vi "wheel velocities.vi"(6 "Track Width":dbl, 11 "Path Data":T1={"Path"=[], "Target Velocities"=[], "Robot Location"=[], "Relative Robot Angle (rad)"=0.0, "Curvature"=0.0, "Lookahead Point"=[3064.399009129367, 18229.833030071386], "Lookahead Index"=8.422809037111724, "Closest Point"=[], "Closest Point Index"=0, "Left Velocity"=0.0, "Right Velocity"=0.0, "Left Encoder Vel"=0, "Right Encoder Vel"=0, "Left Encoder Pos"=0, "Right Encoder Pos"=0, "Inital Robot Angle (deg)"=0.0}) -> (3 "Path Data":T1={"Path"=[], "Target Velocities"=[], "Robot Location"=[], "Relative Robot Angle (rad)"=0.0, "Curvature"=0.0, "Lookahead Point"=[3064.399009129367, 18229.833030071386], "Lookahead Index"=8.422809037111724, "Closest Point"=[], "Closest Point Index"=0, "Left Velocity"=0.0, "Right Velocity"=0.0, "Left Encoder Vel"=0, "Right Encoder Vel"=0, "Left Encoder Pos"=0, "Right Encoder Pos"=0, "Inital Robot Angle (deg)"=0.0})   [LabVIEW 2018]
uses:
  path data.ctl
panel:
  out "Right Velocity":dbl
  out "Left Velocity":dbl
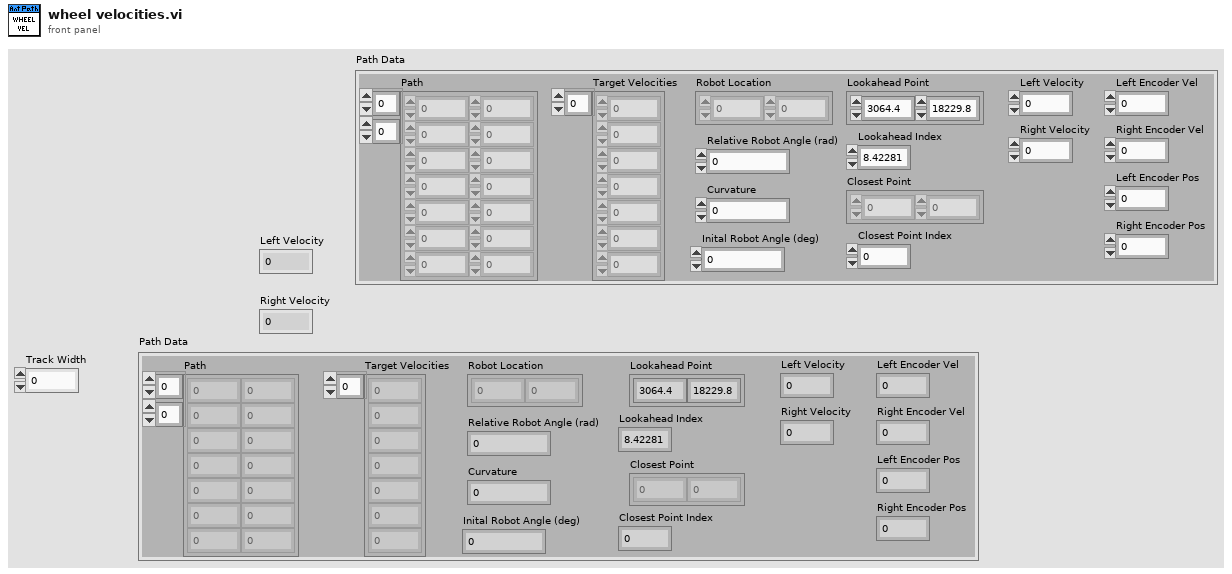
[diagram p1: front panel]
types:
  T1 = typedef "path data.ctl" = cluster{"Path":dbl[][], "Target Velocities":dbl[], "Robot Location":dbl[], "Relative Robot Angle (rad)":dbl, "Curvature":dbl, "Lookahead Point":dbl[], "Lookahead Index":dbl, "Closest Point":dbl[], "Closest Point Index":i32, "Left Velocity":dbl, "Right Velocity":dbl, "Left Encoder Vel":i32, "Right Encoder Vel":i32, "Left Encoder Pos":i32, "Right Encoder Pos":i32, "Inital Robot Angle (deg)":dbl}
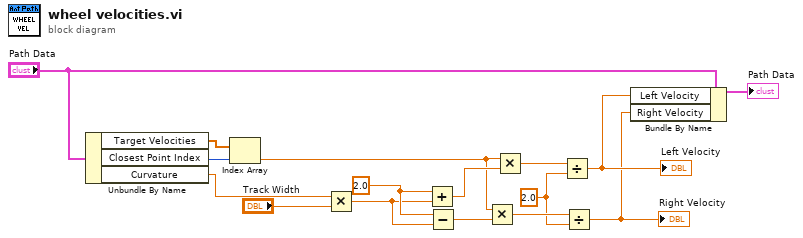
[diagram p0: block diagram]
diagram:
  w9 = 2.0 ("x")
  w15 = 2.0 ("x")
  n1 = Unbundle By Name("Path Data") -> ("Target Velocities"=w3:dbl[], "Closest Point Index"=w4:i32, "Curvature"=w1:dbl)
  n2 = Index Array(array=w3, index=w4) -> (element=w2:dbl)
  n3 = Multiply(x=w1, y="Track Width") -> (x*y=w14:dbl)
  n4 = Add(x=w15, y=w14) -> (x+y=w11:dbl)
  n5 = Subtract(x=w15, y=w14) -> (x-y=w10:dbl)
  n6 = Multiply(x=w2, y=w10) -> (x*y=w12:dbl)
  n7 = Multiply(x=w2, y=w11) -> (x*y=w13:dbl)
  n8 = Divide(x=w13, y=w9) -> (x/y=w6:dbl)
  "Left Velocity" <- w6
  n9 = Divide(x=w12, y=w9) -> (x/y=w5:dbl)
  "Right Velocity" <- w5
  n10 = Bundle By Name(cluster="Path Data", "Left Velocity"=w6, "Right Velocity"=w5) -> (→"Path Data":T1)
